vi "Digital Burst Pattern and Capture.vi"(5 "Published Data Id":string="BoolValid", 6 "Register Data":string[](array[string]), 7 "Pattern Names":string[](array[string]), 9 "CaptureWaveform name":string, 10 "Pin Names":string[](array[string]), 11 "Semiconductor Module Context":T1) -> (0 "error out":errorcluster, 3 "Capture Data":u32[](array[numeric]))   [LabVIEW 2014]
uses:
  <vilib>/NI_TestStand_SemiconductorModule/NI_TestStand_Semiconductor_Module.lvlibp/PinMap/General/SemiconductorModuleContext.ctl
  <vilib>/NI_TestStand_SemiconductorModule/NI_TestStand_Semiconductor_Module.lvlibp/PinMap/Digital Pattern/PinsToNIDigitalPatternSessions.vi
  <instrlib>/niDigital/niDigital.llb/niDigital Burst Pattern (Burst Only).vi
  <vilib>/NI_TestStand_SemiconductorModule/NI_TestStand_Semiconductor_Module.lvlibp/PinMap/General/Publish/PublishDataDoubleFunctionalTest.vi
  <vilib>/NI_TestStand_SemiconductorModule/NI_TestStand_Semiconductor_Module.lvlibp
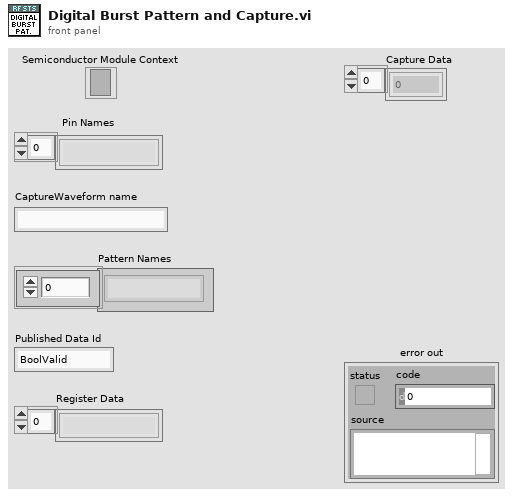
[diagram p1: front panel]
types:
  T1 = typedef "NI_TestStand_Semiconductor_Module.lvlibp/SemiconductorModuleContext.ctl" = refnum<k7>
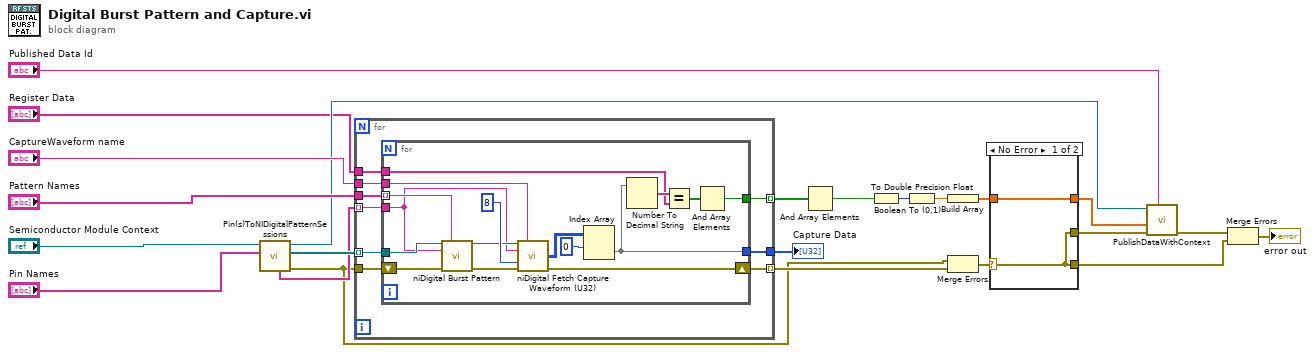
[diagram p0: block diagram]
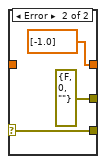
[diagram p2: hidden frame]
diagram:
  n1 = call-poly <vilib>:"Pin(s)ToNIDigitalPatternSessions.vi"("Pins"="Pin Names", "Semiconductor Module Context"="Semiconductor Module Context") -> ("error out"=w14:errorcluster, "Instrument Sessions"=w22:refnum<k15>[], "Semiconductor Module Context Out"=w17:T1, "Site Lists"=w16:string[])  [unwired: 4 in, 2 out]
  n2 = for {
    tunnel: w22 -> [w26] mode=indexing
    tunnel: "Pattern Names" -> [w32]
    tunnel: "CaptureWaveform name" -> [w31]
    tunnel: "Register Data" -> [w29]
    tunnel: [w28] -> w6 mode=indexing
    tunnel: w14 -> [w27]
    tunnel: [w30] -> w15 mode=indexing
    tunnel: w16 -> [w25] mode=indexing
    tunnel: [w24] -> w12
    n3 = for {
      tunnel: w32 -> [w47] mode=indexing
      tunnel: w26 -> [w43]
      tunnel: w31 -> [w44]
      shift-right: [w40] -> w30
      shift-left: w27 -> [w42]
      tunnel: w29 -> [w35]
      tunnel: [w37] -> w28
      tunnel: w25 -> [w39]
      tunnel: [w33] -> w24
      n4 = call-poly <instrlib>:"niDigital Burst Pattern.vi"("instrument handle"=w43, "start label"=w47, "site list"=w39, "error in"=w42) -> ("instrument handle out"=w46:refnum<k15>, "error out"=w45:errorcluster)  [unwired: 10 in]
      n5 = call <instrlib>:"niDigital Fetch Capture Waveform (U32).vi"("instrument handle"=w46, "waveform name"=w44, "site list"=w39, "samples to read"=8, "error in"=w45) -> ("data"=w41:u32[][], "error out"=w40:errorcluster)  [unwired: 8 in, 1 out]
      n6 = Index Array(array=w41, index (row)=0) -> (element=w33:u32[])  [unwired: 1 in]
      n7 = Number To Decimal String(number=w33) -> (decimal integer string=w36:string[])  [unwired: 1 in]
      n8 = Equal?(x=w36, y=w35) -> (x = y?=w34:bool[])
      n9 = And Array Elements(Boolean array=w34) -> (logical AND=w37:bool)
    }
  }
  "Capture Data" <- w12
  n10 = And Array Elements(Boolean array=w6) -> (logical AND=w5:bool)
  n11 = Boolean To (0,1)(Boolean=w5) -> (0, 1=w4:i16)
  n12 = To Double Precision Float(number=w4) -> (double precision float=w3:dbl)
  n13 = Build Array(w3) -> (w2:dbl[])
  n14 = Merge Errors(w14, w15) -> (w11:errorcluster)
  n15 = case shown="No Error" w11 {
    selector: w11 -> [w50 w52]
    tunnel: [w50 errorcluster {"status"=FALSE, "code"=0, "source"=""} ("error IO")] -> w10
    tunnel: [w50 w52] -> w8
    tunnel: w2 -> [w49 _]
    tunnel: [w49 dbl[] [-1.0]] -> w1
    frame No Error {
    }
    frame Error {
    }
  }
  n16 = call-poly <vilib>:"PublishDataWithContext.vi"("Published Data Id"="Published Data Id", "error in (no error)"=w10, "Data In"=w1, "Semiconductor Module Context"=w17) -> ("error out"=w9:errorcluster)  [unwired: 6 in, 1 out]
  n17 = Merge Errors(w9, w8) -> (→"error out":errorcluster)
